vi "escribe_final_equipos.vi"(8 "error in (no error)":errorcluster, 10 "cluster_equipos":T1, 11 "DB in":refnum<class "Base de Datos.lvclass">) -> (0 "error out":errorcluster, 3 "DB out":refnum<class "Base de Datos.lvclass">)   [LabVIEW 2019, in "Base de Datos.lvclass"]
uses:
  Base de Datos.lvclass
  Controles/cluster_equipos.ctl
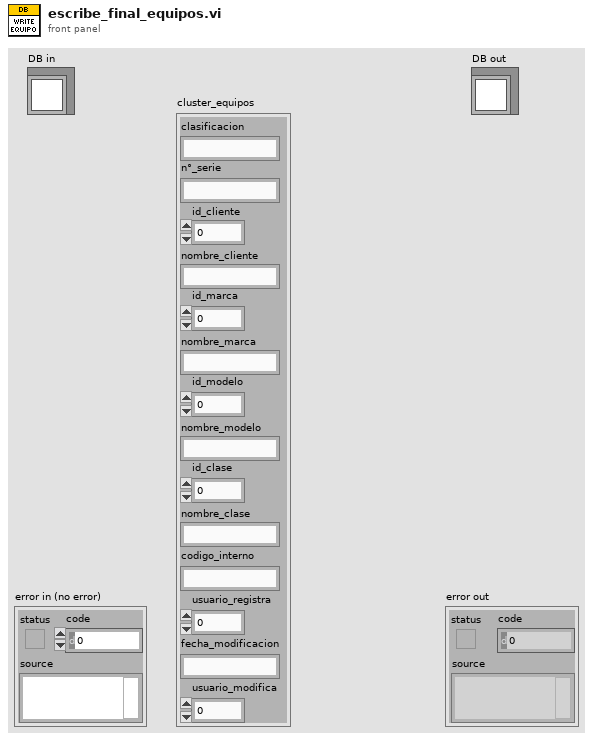
[diagram p1: front panel]
types:
  T1 = typedef "Base de Datos.lvclass/cluster_equipos.ctl" = cluster{"clasificacion":string, "n°_serie":string, "id_cliente":i32, "nombre_cliente":string, "id_marca":i32, "nombre_marca":string, "id_modelo":i32, "nombre_modelo":string, "id_clase":i32, "nombre_clase":string, "codigo_interno":string, "usuario_registra":i32, "fecha_modificacion":string, "usuario_modifica":i32}
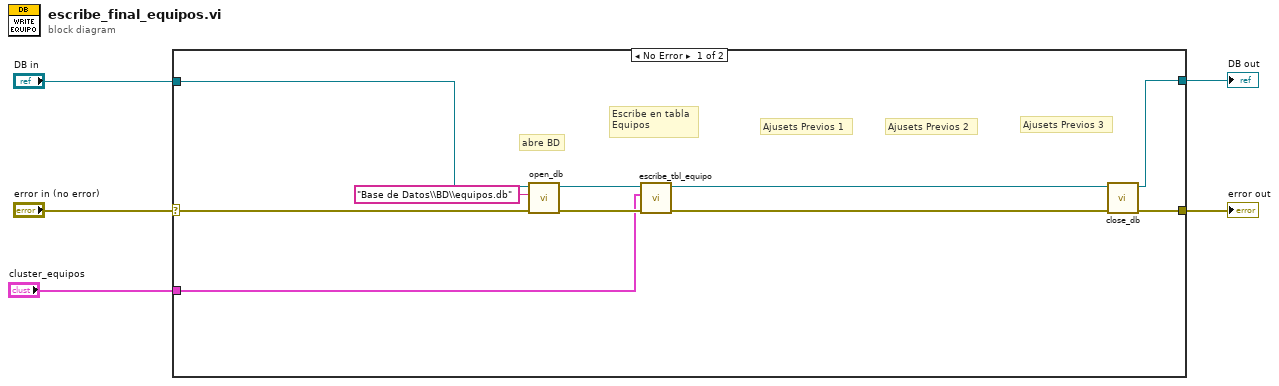
[diagram p0: block diagram]
diagram:
  n1 = case shown="No Error" "error in (no error)" {
    selector: "error in (no error)" -> [w10 w17]
    tunnel: [w11 w17] -> w5
    tunnel: "DB in" -> [w9 w16]
    tunnel: [w8 w16] -> w2
    tunnel: "cluster_equipos" -> [w6 _]
    frame No Error {
      # "abre BD"
      # "Ajusets Previos 3"
      # "Ajusets Previos 2"
      # "Ajusets Previos 1"
      # "Escribe en tabla \nEquipos"
      n2 = call "open_db.vi"("error in (no error)"=w10, 10:"Base de Datos\\BD\\equipos.db" ("BD"), "DB in"=w9) -> ("error out"=w14:errorcluster, "DB out"=w15:refnum<class "Base de Datos.lvclass">)  [unwired: 7 in]
      n3 = call "escribe_tbl_equipo.vi"("error in (no error)"=w14, "cluster_equipos"=w6, "DB in"=w15) -> ("error out"=w12:errorcluster, "object out"=w13:refnum<class "Base de Datos.lvclass">)  [unwired: 7 in]
      n4 = call "close_db.vi"("error in (no error)"=w12, "BD in"=w13) -> ("error out"=w11:errorcluster, "BD out"=w8:refnum<class "Base de Datos.lvclass">)  [unwired: 8 in]
    }
    frame Error {
    }
  }
  "error out" <- w5
  "DB out" <- w2
